vi "RX.vi"(7 "Timeout (10000)":i32=10000, 8 "error in (no error)":errorcluster, 9 "Transaction Notifier":refnum<notifier>, 10 "Transaction LUT in":refnum<data-value>, 11 "ADU in":refnum<class "MB_ADU_TCP.lvclass">) -> (0 "error out":errorcluster, 1 "PDU_resp":T1={"Function Code"=1, "Data"=[], "RTU_DataBytes"=0}, 2 "Transaction LUT out":refnum<data-value>, 3 "ADU out":refnum<class "MB_ADU_TCP.lvclass">)   [LabVIEW 2023, in "Jiaxin_Stepper_Controller.lvlib" / "MB Master.lvlib" / "MB_Master_TCP.lvclass"]
uses:
  MB_Master_TCP.lvclass
  MB_ADU_TCP/MB_ADU_TCP.lvclass
  MB_PDU/MB_PDU_Cluster.ctl
  MB_ADU_TCP/MB_ADU_TCP.lvclass/MB_ADU_TCP.ctl
  MB_ADU_TCP/Read Transaction ID.vi
  MB Master.lvlib
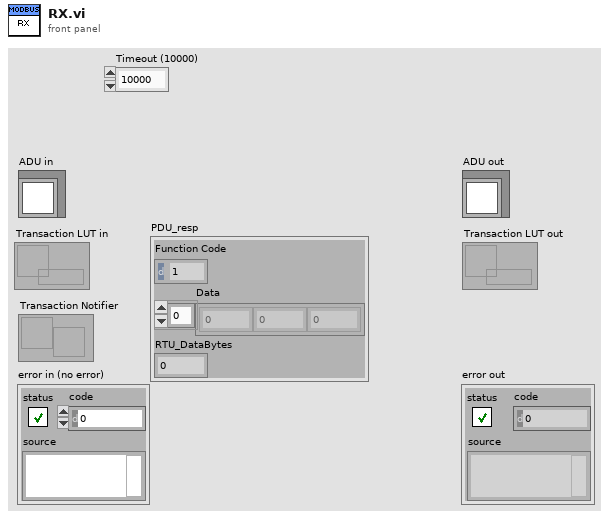
[diagram p1: front panel]
types:
  T1 = typedef "Jiaxin_Stepper_Controller.lvlib/MB Master.lvlib/MB_PDU_Cluster.ctl" = cluster{"Function Code":u8, "Data":u8[], "RTU_DataBytes":i32}
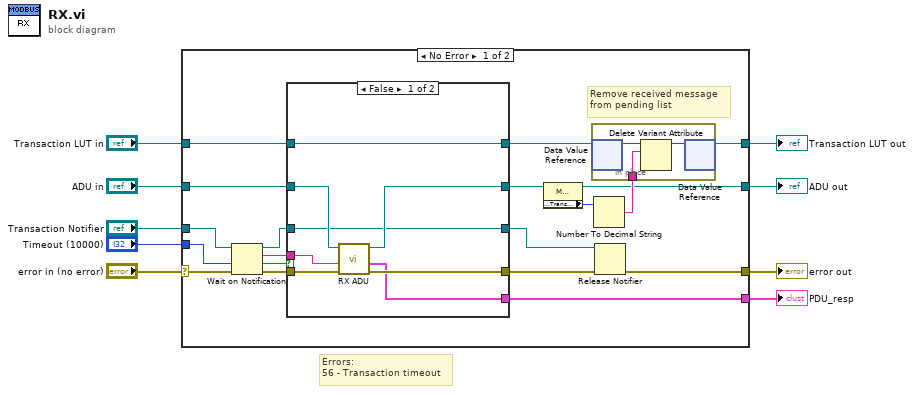
[diagram p0: block diagram]
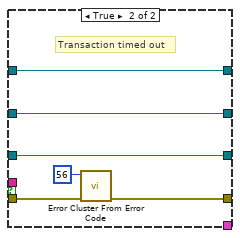
[diagram p2: hidden frame]
diagram:
  # "Errors:\n56 - Transaction timeout"
  n1 = case shown="No Error" "error in (no error)" {
    selector: "error in (no error)" -> [w24 w48]
    tunnel: [w17 w48] -> w8
    tunnel: "Transaction LUT in" -> [w20 w47]
    tunnel: [w10 w47] -> w6
    tunnel: "ADU in" -> [w26 w46]
    tunnel: [w12 w46] -> w4
    tunnel: "Transaction Notifier" -> [w25 _]
    tunnel: [w23 _] -> w2
    tunnel: "Timeout (10000)" -> [w22 _]
    frame No Error {
      # "Remove received message\nfrom pending list"
      n2 = Wait on Notification(notifier=w25, timeout in ms (-1)=w22, error in (no error)=w24) -> (notifier out=w19:refnum<notifier>, notification=w28:string, timed out?=w21:bool, error out=w27:errorcluster)  [unwired: 1 in]
      n3 = case shown="False" w21 {
        tunnel: w28 -> [w39 _]
        tunnel: [w38 w43] -> w18
        tunnel: w27 -> [w37 w44]
        tunnel: w26 -> [w36 w40]
        tunnel: [w35 w40] -> w13
        tunnel: [w34 _] -> w23
        tunnel: w20 -> [w32 w41]
        tunnel: w19 -> [w33 w45]
        tunnel: [w32 w41] -> w11
        tunnel: [w33 w45] -> w16
        frame False {
          n4 = call "RX ADU.vi"("error in (no error)"=w37, "RX Data"=w39, "MB_ADU_TCP in"=w36) -> ("error out"=w38:errorcluster, "PDU_resp"=w34:T1, "MB_ADU_TCP out"=w35:refnum<class "MB_ADU_TCP.lvclass">)  [unwired: 6 in]
        }
        frame True {
          # "Transaction timed out"
          n5 = call <vilib>:"Error Cluster From Error Code.vi"("error in (no error)"=w44, "error code (0)"=56) -> ("error out"=w43:errorcluster)  [unwired: 7 in]
        }
      }
      n6 = property class="MB_ADU_TCP"(reference=w13) -> (reference out=w12:refnum<class "MB_ADU_TCP.lvclass">, "Properties:Transaction ID"=w15:u16)  [unwired: 1 in, 1 out]
      n7 = Number To Decimal String(number=w15) -> (decimal integer string=w14:string)  [unwired: 1 in]
      n8 = in-place {
        in-place-border: w14 -> [w30]
        n9 = in-place-dvr #1(w11) -> (w29:variant)  [unwired: 1 out]
        n10 = Delete Variant Attribute(6:w30, 7:w29) -> (3:w31:variant)  [unwired: 1 in, 2 out]
        n11 = in-place-dvr #1(w31) -> (w10:refnum<data-value>)  [unwired: 1 out]
      }
      n12 = Release Notifier(notifier=w16, error in (no error)=w18) -> (error out=w17:errorcluster)  [unwired: 1 in, 2 out]
    }
    frame Error {
    }
  }
  "error out" <- w8
  "Transaction LUT out" <- w6
  "ADU out" <- w4
  "PDU_resp" <- w2
